vi "Top Level FPGA_w8LED.vi"() -> ()   [LabVIEW 2012]
uses:
  <vilib>/Platform/TimedLoop/XDataNode/timing_clust.ctl
  <vilib>/Platform/TimedLoop/XDataNode/nitl_modes.ctl
  <vilib>/Platform/TimedLoop/XDataNode/wakeup.ctl
  <vilib>/rvi/DataTransferAndStorage/Container/Common/niFpgaContainerMetaDataKey.ctl
  <vilib>/rvi/DataTransferAndStorage/Container/Common/niFpgaContainerState.ctl
  <vilib>/rvi/DataTransferAndStorage/Container/Common/niFpgaDataTypeControl.ctl
  <vilib>/rvi/DataTransferAndStorage/Container/Common/niFpgaContainerImplementationControl.ctl
  <vilib>/rvi/DataTransferAndStorage/Container/Common/niFpgaContainerArbitrationOptionsControl.ctl
  <vilib>/rvi/DataTransferAndStorage/Container/Common/niFpgaTransferTypeControl.ctl
  <vilib>/rvi/DataTransferAndStorage/Container/Common/niFpgaContainerInitializationParameters.ctl
  <vilib>/rvi/Memory/Memory_Types/niFpgaMemoryInterfaceConfiguration.ctl
  <vilib>/rvi/FIFO/Fifo_Types/niFpgaFifoControlLogicControl.ctl
  <vilib>/rvi/eio/common/nirviEmuTemplateMethod_errors.vi
  <vilib>/rvi/FIFO/Fifo_Resource/nirvififoEmulationSetSize.vi
  <vilib>/rvi/DataTransferAndStorage/Container/Common/niFpgaContainerGetUniqueNameForEmu.vi
  <vilib>/rvi/Emulation/niFpgaSctlEmulationRegisterWithScheduler.vi
  <vilib>/rvi/Emulation/niFpgaSctlEmulationScheduler.vi
  <vilib>/rvi/Emulation/niFpgaSctlEmulationFifoFullMgr.vi
  <vilib>/rvi/errors/niFpgaSetErrorForExecOnDevCompSimple.vi
  <vilib>/rvi/eio/common/nirviEmuReportErrorAndStop.vi
  <vilib>/rvi/Memory/Memory_Emulation/nirvimemoryEmulationManagerCache_GetValue.vi
  <vilib>/rvi/Memory/Memory_Emulation/niFpgaMemoryEmulationValidateCache.vi
  <vilib>/rvi/Memory/Memory_Emulation/nirvimemoryEmulationManagerCache_InsertValue.vi
  <vilib>/rvi/Memory/Memory_Emulation/nirvimemoryEmulationManagerCache_SetValue.vi
  <vilib>/rvi/Emulation/niFpgaSctlEmulationResourceMgr.vi
  <vilib>/rvi/Memory/Memory_Emulation/niFpgaMemoryEmulationCacheClearOnFirstRun.vi
  <vilib>/rvi/Memory/Memory_Emulation/nirvimemoryEmulationManagerCache_MakeExclusive.vi
  <vilib>/rvi/Memory/Memory_Emulation/nirvimemoryEmulationManagerCache_ReleaseExclusive.vi
  <vilib>/Utility/error.llb/Clear Errors.vi
  <vilib>/rvi/DataTransferAndStorage/Container/Common/niFpgaContainerSetEmuInfo.vi
  <vilib>/eio/EIONode/EIONode.xnode
  <vilib>/Platform/TimedLoop/XDataNode/XDataNode.xnode
  <vilib>/rvi/DataTransferAndStorage/Container/XNode/niFpgaContainer.xnode
  <vilib>/rvi/FIFO/Fifo_Resource/nirvififoEmulationClear.vi
  <vilib>/rvi/FIFO/Fifo_Resource/nirvififoEmulationRead.vi
  <vilib>/rvi/DataTransferAndStorage/Register/Emulation/niFpgaRegisterEmulation.vi
  <vilib>/rvi/Memory/Memory_Emulation/nirvimemoryEmulation.vi
  <vilib>/rvi/FIFO/Fifo_Resource/nirvififoEmulationWrite.vi
  <vilib>/rvi/LocalResourceManager/LocalResourceManager.xnode
  <vilib>/Platform/TimedLoop/XDataNode/XDNodeRunTimeDep.lvlib
panel:
  out "IO Module\\ADC Error A":bool
  out "IO Module\\ADC Error B":bool
  out "IO Module\\Pll Unlocked":bool
  out "Exited cleanly?":bool
  in  "Stop FPGA and exit":bool
  in  "Record Size only data":u32=95
  in  "show_trigger_position_for_debugging":bool
  out "DMA FIFO Timed Out?":bool
  in  "circular buffer length":u32=1000
  in  "location":i16(ring) items=["Purdue", "NIKHEF", "Zurich", "???"]
  in  "Trigger 0":i16=4000
  in  "Trigger 1":i16=4000
  in  "Trigger 2":i16=4000
  in  "Trigger 3":i16=4000
  in  "Trigger 4":i16=4000
  in  "Trigger 5":i16=4000
  in  "Trigger 6":i16=4000
  in  "Trigger 7":i16=4000
  in  "# of pretrigger":u32=20
  in  "initial value":u64
  in  "channel 0 on/off":bool
  in  "channel 2 on/off":bool
  in  "channel 1 on/off":bool
  in  "channel 3 on/off":bool
  in  "channel 4 on/off":bool
  in  "channel 5 on/off":bool
  in  "channel 6 on/off":bool
  in  "channel 7 on/off":bool
  out "Is Channel 0 Test Pulse?":bool
  in  "Testpulse duration (20 ns ticks)":u32=1
  in  "Testpulse Separation (20 ns ticks)":u32=500
  in  "Testpulse Time Delay (20 ns ticks)":u32=15
  out "Timestamp":u64
  out "Is Channel 1 Test Pulse?":bool
  in  "Testpulser On/Off":bool
  out "Is Channel 2 Test Pulse?":bool
  out "Is Channel 3 Test Pulse?":bool
  out "Is Channel 4 Test Pulse?":bool
  out "Is Channel 5 Test Pulse?":bool
  out "Is Channel 6 Test Pulse?":bool
  out "Is Channel 7 Test Pulse?":bool
  out "Init Done":bool
  out "Initialize Flush DMA FIFO":bool
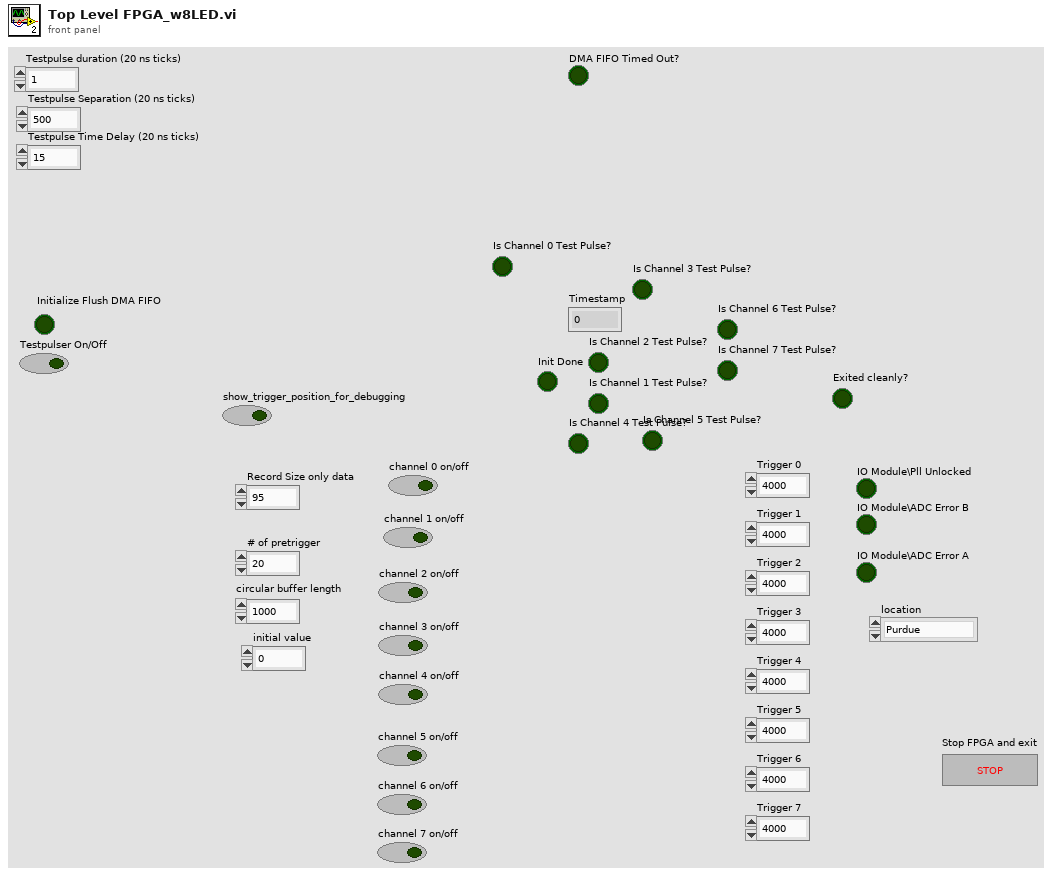
[diagram p1: front panel]
types:
  T1 = typedef "XDNodeRunTimeDep.lvlib/timing_clust.ctl" = cluster{"Expected End [f-1]":u64, "Actual End [f-1]":u64, "Finished Late? [f-1]":bool, "Expected End [i-1]":u64, "Actual End [i-1]":u64, "Finished Late? [i-1]":bool, "Expected Start [i]":u64, "Actual Start [i]":u64, "Expected Start [f]":u64, "Actual Start [f]":u64, "Source Name":string, "Structure Name":string, "Period":i64, "Deadline":i64, "Offset":i64, "Start":i64, "Priority":i32, "Timeout":i32, "Mode":T2, "Wakeup Reason":T3, "Error":errorcluster, "Source Type":string, "Secondary Source Type":string, "Global End Time":u64, "Global Start Time":u64, "Frame Duration":u64, "Iteration Duration":u64, "Assigned CPU":i32, "I/O Scan Engine Mode":u32}
  T2 = typedef "XDNodeRunTimeDep.lvlib/nitl_modes.ctl" = enum32{"No Change", "Process missed periods, maintain original phase", "Discard missed periods, maintain original phase", "Process missed periods, ignore original phase", "Discard missed periods, ignore original phase"}
  T3 = typedef "XDNodeRunTimeDep.lvlib/wakeup.ctl" = enum32{"Normal", "Aborted", "Asynchronous wakeup", "Timing source error", "Timed loop error", "Timeout"}
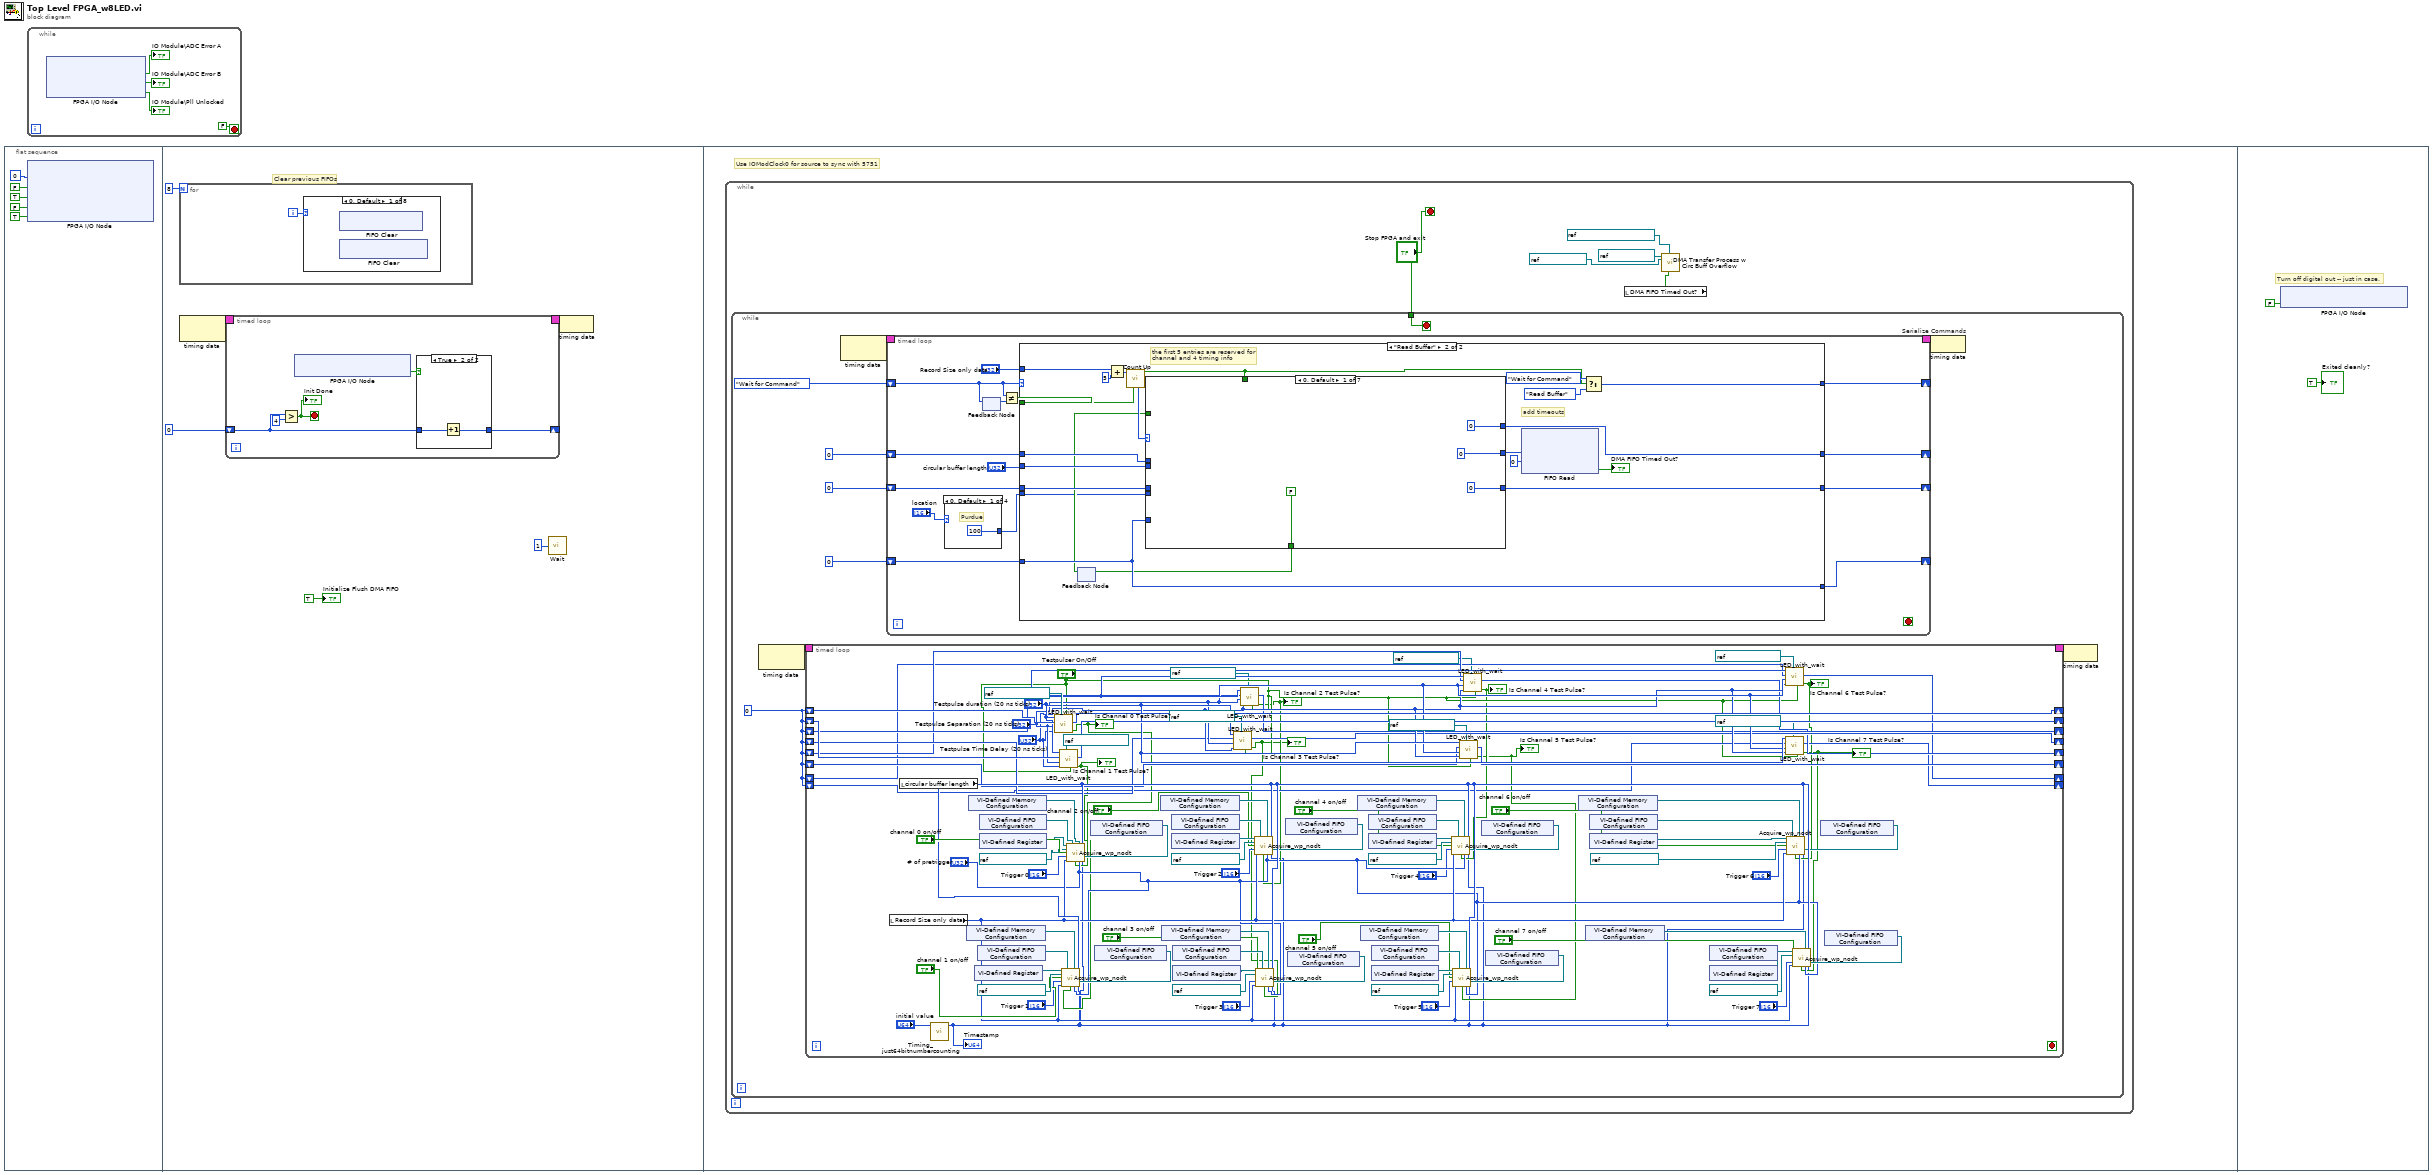
[diagram p0: block diagram]
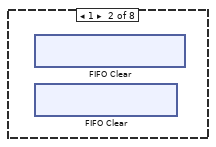
[diagram p2: hidden frame]
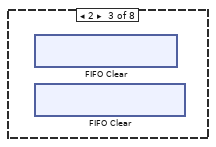
[diagram p3: hidden frame]
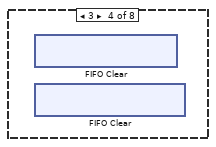
[diagram p4: hidden frame]
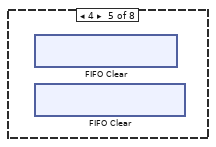
[diagram p5: hidden frame]
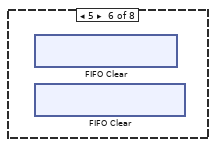
[diagram p6: hidden frame]
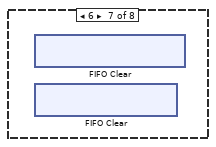
[diagram p7: hidden frame]
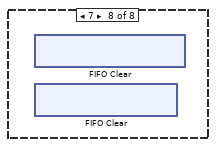
[diagram p8: hidden frame]
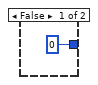
[diagram p9: hidden frame]
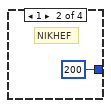
[diagram p10: hidden frame]
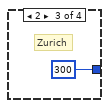
[diagram p11: hidden frame]
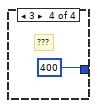
[diagram p12: hidden frame]
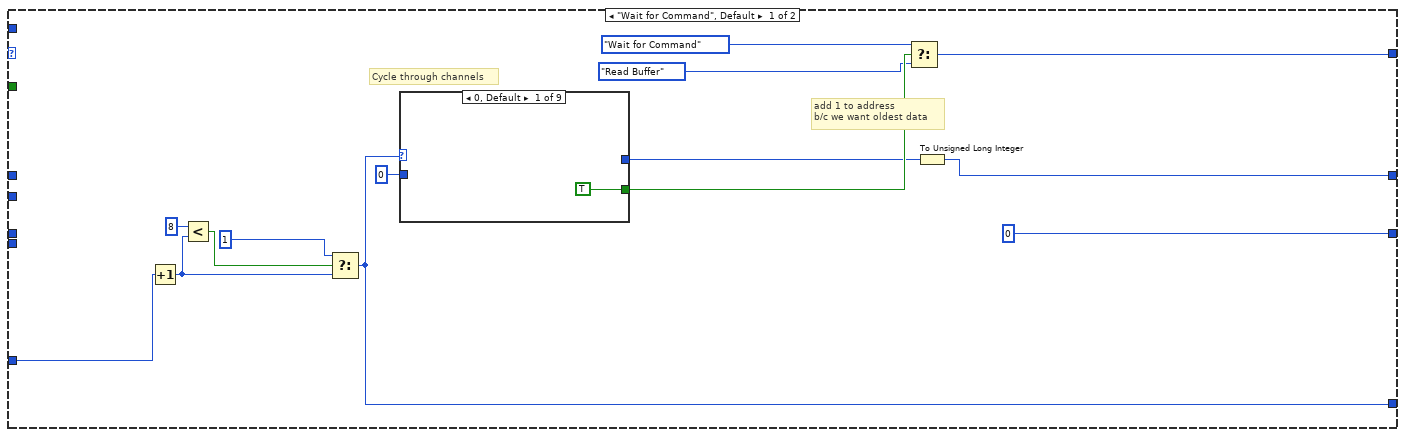
[diagram p13: hidden frame]
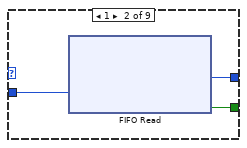
[diagram p14: hidden frame]
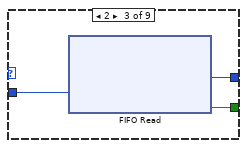
[diagram p15: hidden frame]
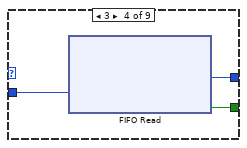
[diagram p16: hidden frame]
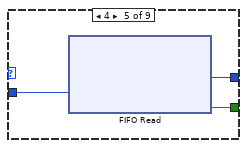
[diagram p17: hidden frame]
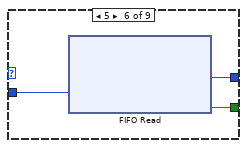
[diagram p18: hidden frame]
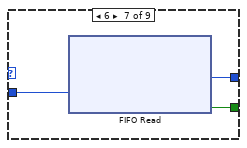
[diagram p19: hidden frame]
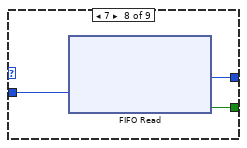
[diagram p20: hidden frame]
diagram:
  n1 = flat-sequence {
    frame #0 {
      n2 = xnode "FPGA I/O Node"("IO Module\\Sample Clock Select"=u8 0 ("IO Module\\Sample Clock Select"), "IO Module\\Force Initialization"=FALSE ("IO Module\\Force Initialization"), "IO Module\\Force Initialization"=TRUE ("IO Module\\Force Initialization"), "IO Module\\Force Initialization"=FALSE ("IO Module\\Force Initialization"), "IO Module\\Digital Output Enable"=TRUE ("IO Module\\Digital Output Enable")) -> ()  [unwired: 5 in, 5 out]
    }
    frame #1 {
      # "Clear previous FIFOs"
      n3 = for {
        N: 8 -> [_]
        i -> [w12]
        n4 = case shown="0, Default" w12 {
          frame 0, Default {
            n5 = xnode ("FIFO Clear")() -> ()  [unwired: 1 in, 1 out]
            n6 = xnode ("FIFO Clear")() -> ()  [unwired: 1 in, 1 out]
          }
          frame 1 {
            n7 = xnode ("FIFO Clear")() -> ()  [unwired: 1 in, 1 out]
            n8 = xnode ("FIFO Clear")() -> ()  [unwired: 1 in, 1 out]
          }
          frame 2 {
            n9 = xnode ("FIFO Clear")() -> ()  [unwired: 1 in, 1 out]
            n10 = xnode ("FIFO Clear")() -> ()  [unwired: 1 in, 1 out]
          }
          frame 3 {
            n11 = xnode ("FIFO Clear")() -> ()  [unwired: 1 in, 1 out]
            n12 = xnode ("FIFO Clear")() -> ()  [unwired: 1 in, 1 out]
          }
          frame 4 {
            n13 = xnode ("FIFO Clear")() -> ()  [unwired: 1 in, 1 out]
            n14 = xnode ("FIFO Clear")() -> ()  [unwired: 1 in, 1 out]
          }
          frame 5 {
            n15 = xnode ("FIFO Clear")() -> ()  [unwired: 1 in, 1 out]
            n16 = xnode ("FIFO Clear")() -> ()  [unwired: 1 in, 1 out]
          }
          frame 6 {
            n17 = xnode ("FIFO Clear")() -> ()  [unwired: 1 in, 1 out]
            n18 = xnode ("FIFO Clear")() -> ()  [unwired: 1 in, 1 out]
          }
          frame 7 {
            n19 = xnode ("FIFO Clear")() -> ()  [unwired: 1 in, 1 out]
            n20 = xnode ("FIFO Clear")() -> ()  [unwired: 1 in, 1 out]
          }
        }
      }
      n21 = node-c288() -> (w11:T1)  [unwired: 1 in]
      n22 = timed-loop {
        shift-right: [w16] -> _
        shift-left: u16 0 -> [w15]
        timing: w11 -> [_]
        timing-out: [_] -> w10
        stop <- w13 stop-if-true
        n23 = Greater?(x=w15, y=u16 4) -> (0:w13:bool)
        "Init Done" <- w13
        n24 = xnode "FPGA I/O Node"() -> ("IO Module\\Initialization Done"=w17:bool)  [unwired: 1 in, 1 out]
        n25 = case shown="True" w17 {
          tunnel: [u16 0 w20] -> w16
          tunnel: w15 -> [_ w19]
          frame False {
          }
          frame True {
            n26 = Increment(x=w19) -> (x+1=w20:u16)
          }
        }
      }
      n27 = call "Wait"("Count(mSec)"=u32 1) -> ()  [unwired: 1 out]
      n28 = node-c288(w10) -> ()
      "Initialize Flush DMA FIFO" <- TRUE ("Initialize Flush DMA FIFO")
    }
    frame #2 {
      # "Use IOModClock0 for source to sync with 5751"
      n29 = while {
        stop <- "Stop FPGA and exit" stop-if-true
        n30 = while {
          tunnel: "Stop FPGA and exit" -> [w31]
          stop <- w31 stop-if-true
          w30 = u64 0 ("Total number of pulses sent")
          n31 = node-c288() -> (w37:T1)  [unwired: 1 in]
          n32 = timed-loop {
            timing: w37 -> [_]
            timing-out: [_] -> w36
            shift-right: [w94] -> _
            shift-left: w30 -> [w95]
            shift-right: [w90] -> _
            shift-left: w30 -> [w91]
            shift-right: [w83] -> _
            shift-left: w30 -> [w84]
            shift-right: [w82] -> _
            shift-left: w30 -> [w77]
            shift-right: [w81] -> _
            shift-left: w30 -> [w76]
            shift-right: [w80] -> _
            shift-left: w30 -> [w75]
            shift-right: [w79] -> _
            shift-left: w30 -> [w74]
            shift-right: [w78] -> _
            shift-left: w30 -> [w73]
            stop <- _ stop-if-true
            n33 = local read "Record Size only data"() -> (w96:u32)
            n34 = local read "circular buffer length"() -> (w97:u32)
            n35 = call "Timing_just64bitnumbercounting.vi"("initial value"="initial value") -> ("x+1"=w40:u64)  [unwired: 10 in]
            "Timestamp" <- w40
            n36 = xnode "VI-Defined Memory Configuration"() -> ("Memory Out"=w136:refnum<k21>)
            n37 = xnode "VI-Defined Memory Configuration"() -> ("Memory Out"=w98:refnum<k21>)
            n38 = xnode "VI-Defined Register"() -> ("Register Out"=w88:refnum<k21>)
            n39 = xnode "VI-Defined FIFO Configuration"() -> ("FIFO Out"=w135:refnum<k21>)
            n40 = xnode "VI-Defined FIFO Configuration"() -> ("FIFO Out"=w99:refnum<k21>)
            n41 = xnode "VI-Defined Register"() -> ("Register Out"=w89:refnum<k21>)
            n42 = call "LED_with_wait.vi"("Testpulser On/Off"="Testpulser On/Off", "FPGA I/O In"=refnum<k21> "IO Module\\D0 0", "Testpulse Time Delay (20 ns ticks)"="Testpulse Time Delay (20 ns ticks)", "Testpulse Separation (20 ns ticks)"="Testpulse Separation (20 ns ticks)", "Total number of pulses input"=w95, "Testpulse duration (20 ns ticks)"="Testpulse duration (20 ns ticks)") -> ("Is Test Pulse?"=w42:bool, "Total number of pulses sent"=w94:u64)  [unwired: 4 in]
            "Is Channel 0 Test Pulse?" <- w42
            n43 = call "LED_with_wait.vi"("Testpulser On/Off"="Testpulser On/Off", "FPGA I/O In"=refnum<k21> "IO Module\\D0 1", "Testpulse Time Delay (20 ns ticks)"="Testpulse Time Delay (20 ns ticks)", "Testpulse Separation (20 ns ticks)"="Testpulse Separation (20 ns ticks)", "Total number of pulses input"=w91, "Testpulse duration (20 ns ticks)"="Testpulse duration (20 ns ticks)") -> ("Is Test Pulse?"=w41:bool, "Total number of pulses sent"=w90:u64)  [unwired: 4 in]
            "Is Channel 1 Test Pulse?" <- w41
            n44 = xnode "VI-Defined FIFO Configuration"() -> ("FIFO Out"=w65:refnum<k21>)
            n45 = call "Acquire_wp_nodt.vi"("Ch Armed Reg"=w89, "Command FIFO"=w99, "Circular Buffer Mem"=w98, "circular buffer length"=w97, "FPGA I/O In"=refnum<k21> "IO Module\\AI A0", "channel on/off"="channel 0 on/off", "Trigger"="Trigger 0", "Timing FIFO"=w65, "Samples to Acquire"=w96, "Is Test Pulse?"=w42, "# of pretrigger"="# of pretrigger", "timing"=w40) -> ()  [unwired: 4 in]
            n46 = xnode "VI-Defined FIFO Configuration"() -> ("FIFO Out"=w58:refnum<k21>)
            n47 = call "Acquire_wp_nodt.vi"("Ch Armed Reg"=w88, "Command FIFO"=w135, "Circular Buffer Mem"=w136, "circular buffer length"=w97, "FPGA I/O In"=refnum<k21> "IO Module\\AI A1", "channel on/off"="channel 1 on/off", "Trigger"="Trigger 1", "Timing FIFO"=w58, "Samples to Acquire"=w96, "Is Test Pulse?"=w41, "# of pretrigger"="# of pretrigger", "timing"=w40) -> ()  [unwired: 4 in]
            n48 = xnode "VI-Defined Memory Configuration"() -> ("Memory Out"=w132:refnum<k21>)
            n49 = xnode "VI-Defined Memory Configuration"() -> ("Memory Out"=w133:refnum<k21>)
            n50 = xnode "VI-Defined FIFO Configuration"() -> ("FIFO Out"=w131:refnum<k21>)
            n51 = xnode "VI-Defined Register"() -> ("Register Out"=w119:refnum<k21>)
            n52 = xnode "VI-Defined FIFO Configuration"() -> ("FIFO Out"=w134:refnum<k21>)
            n53 = xnode "VI-Defined Register"() -> ("Register Out"=w121:refnum<k21>)
            n54 = call "LED_with_wait.vi"("Testpulser On/Off"="Testpulser On/Off", "FPGA I/O In"=refnum<k21> "IO Module\\D0 3", "Testpulse Time Delay (20 ns ticks)"="Testpulse Time Delay (20 ns ticks)", "Testpulse Separation (20 ns ticks)"="Testpulse Separation (20 ns ticks)", "Total number of pulses input"=w77, "Testpulse duration (20 ns ticks)"="Testpulse duration (20 ns ticks)") -> ("Is Test Pulse?"=w43:bool, "Total number of pulses sent"=w82:u64)  [unwired: 4 in]
            "Is Channel 3 Test Pulse?" <- w43
            n55 = call "LED_with_wait.vi"("Testpulser On/Off"="Testpulser On/Off", "FPGA I/O In"=refnum<k21> "IO Module\\D0 2", "Testpulse Time Delay (20 ns ticks)"="Testpulse Time Delay (20 ns ticks)", "Testpulse Separation (20 ns ticks)"="Testpulse Separation (20 ns ticks)", "Total number of pulses input"=w84, "Testpulse duration (20 ns ticks)"="Testpulse duration (20 ns ticks)") -> ("Is Test Pulse?"=w44:bool, "Total number of pulses sent"=w83:u64)  [unwired: 4 in]
            "Is Channel 2 Test Pulse?" <- w44
            n56 = xnode "VI-Defined FIFO Configuration"() -> ("FIFO Out"=w64:refnum<k21>)
            n57 = call "Acquire_wp_nodt.vi"("Ch Armed Reg"=w119, "Command FIFO"=w131, "Circular Buffer Mem"=w132, "circular buffer length"=w97, "FPGA I/O In"=refnum<k21> "IO Module\\AI A2", "channel on/off"="channel 2 on/off", "Trigger"="Trigger 2", "Timing FIFO"=w64, "Samples to Acquire"=w96, "Is Test Pulse?"=w44, "# of pretrigger"="# of pretrigger", "timing"=w40) -> ()  [unwired: 4 in]
            n58 = xnode "VI-Defined FIFO Configuration"() -> ("FIFO Out"=w59:refnum<k21>)
            n59 = call "Acquire_wp_nodt.vi"("Ch Armed Reg"=w121, "Command FIFO"=w134, "Circular Buffer Mem"=w133, "circular buffer length"=w97, "FPGA I/O In"=refnum<k21> "IO Module\\AI A3", "channel on/off"="channel 3 on/off", "Trigger"="Trigger 3", "Timing FIFO"=w59, "Samples to Acquire"=w96, "Is Test Pulse?"=w43, "# of pretrigger"="# of pretrigger", "timing"=w40) -> ()  [unwired: 4 in]
            n60 = xnode "VI-Defined Memory Configuration"() -> ("Memory Out"=w124:refnum<k21>)
            n61 = xnode "VI-Defined Memory Configuration"() -> ("Memory Out"=w125:refnum<k21>)
            n62 = xnode "VI-Defined Register"() -> ("Register Out"=w113:refnum<k21>)
            n63 = xnode "VI-Defined FIFO Configuration"() -> ("FIFO Out"=w123:refnum<k21>)
            n64 = xnode "VI-Defined FIFO Configuration"() -> ("FIFO Out"=w126:refnum<k21>)
            n65 = xnode "VI-Defined Register"() -> ("Register Out"=w117:refnum<k21>)
            n66 = call "LED_with_wait.vi"("Testpulser On/Off"="Testpulser On/Off", "FPGA I/O In"=refnum<k21> "IO Module\\D0 5", "Testpulse Time Delay (20 ns ticks)"="Testpulse Time Delay (20 ns ticks)", "Testpulse Separation (20 ns ticks)"="Testpulse Separation (20 ns ticks)", "Total number of pulses input"=w75, "Testpulse duration (20 ns ticks)"="Testpulse duration (20 ns ticks)") -> ("Is Test Pulse?"=w45:bool, "Total number of pulses sent"=w80:u64)  [unwired: 4 in]
            "Is Channel 5 Test Pulse?" <- w45
            n67 = call "LED_with_wait.vi"("Testpulser On/Off"="Testpulser On/Off", "FPGA I/O In"=refnum<k21> "IO Module\\D0 4", "Testpulse Time Delay (20 ns ticks)"="Testpulse Time Delay (20 ns ticks)", "Testpulse Separation (20 ns ticks)"="Testpulse Separation (20 ns ticks)", "Total number of pulses input"=w76, "Testpulse duration (20 ns ticks)"="Testpulse duration (20 ns ticks)") -> ("Is Test Pulse?"=w46:bool, "Total number of pulses sent"=w81:u64)  [unwired: 4 in]
            "Is Channel 4 Test Pulse?" <- w46
            n68 = xnode "VI-Defined FIFO Configuration"() -> ("FIFO Out"=w63:refnum<k21>)
            n69 = call "Acquire_wp_nodt.vi"("Ch Armed Reg"=w113, "Command FIFO"=w123, "Circular Buffer Mem"=w124, "circular buffer length"=w97, "FPGA I/O In"=refnum<k21> "IO Module\\AI A4", "channel on/off"="channel 4 on/off", "Trigger"="Trigger 4", "Timing FIFO"=w63, "Samples to Acquire"=w96, "Is Test Pulse?"=w46, "# of pretrigger"="# of pretrigger", "timing"=w40) -> ()  [unwired: 4 in]
            n70 = xnode "VI-Defined FIFO Configuration"() -> ("FIFO Out"=w60:refnum<k21>)
            n71 = call "Acquire_wp_nodt.vi"("Ch Armed Reg"=w117, "Command FIFO"=w126, "Circular Buffer Mem"=w125, "circular buffer length"=w97, "FPGA I/O In"=refnum<k21> "IO Module\\AI A5", "channel on/off"="channel 5 on/off", "Trigger"="Trigger 5", "Timing FIFO"=w60, "Samples to Acquire"=w96, "Is Test Pulse?"=w45, "# of pretrigger"="# of pretrigger", "timing"=w40) -> ()  [unwired: 4 in]
            n72 = xnode "VI-Defined Memory Configuration"() -> ("Memory Out"=w129:refnum<k21>)
            n73 = xnode "VI-Defined Memory Configuration"() -> ("Memory Out"=w128:refnum<k21>)
            n74 = xnode "VI-Defined FIFO Configuration"() -> ("FIFO Out"=w130:refnum<k21>)
            n75 = xnode "VI-Defined Register"() -> ("Register Out"=w115:refnum<k21>)
            n76 = xnode "VI-Defined FIFO Configuration"() -> ("FIFO Out"=w127:refnum<k21>)
            n77 = xnode "VI-Defined Register"() -> ("Register Out"=w111:refnum<k21>)
            n78 = call "LED_with_wait.vi"("Testpulser On/Off"="Testpulser On/Off", "FPGA I/O In"=refnum<k21> "IO Module\\D0 6", "Testpulse Time Delay (20 ns ticks)"="Testpulse Time Delay (20 ns ticks)", "Testpulse Separation (20 ns ticks)"="Testpulse Separation (20 ns ticks)", "Total number of pulses input"=w74, "Testpulse duration (20 ns ticks)"="Testpulse duration (20 ns ticks)") -> ("Is Test Pulse?"=w48:bool, "Total number of pulses sent"=w79:u64)  [unwired: 4 in]
            "Is Channel 6 Test Pulse?" <- w48
            n79 = call "LED_with_wait.vi"("Testpulser On/Off"="Testpulser On/Off", "FPGA I/O In"=refnum<k21> "IO Module\\D0 7", "Testpulse Time Delay (20 ns ticks)"="Testpulse Time Delay (20 ns ticks)", "Testpulse Separation (20 ns ticks)"="Testpulse Separation (20 ns ticks)", "Total number of pulses input"=w73, "Testpulse duration (20 ns ticks)"="Testpulse duration (20 ns ticks)") -> ("Is Test Pulse?"=w47:bool, "Total number of pulses sent"=w78:u64)  [unwired: 4 in]
            "Is Channel 7 Test Pulse?" <- w47
            n80 = xnode "VI-Defined FIFO Configuration"() -> ("FIFO Out"=w62:refnum<k21>)
            n81 = call "Acquire_wp_nodt.vi"("Ch Armed Reg"=w115, "Command FIFO"=w130, "Circular Buffer Mem"=w129, "circular buffer length"=w97, "FPGA I/O In"=refnum<k21> "IO Module\\AI A6", "channel on/off"="channel 6 on/off", "Trigger"="Trigger 6", "Timing FIFO"=w62, "Samples to Acquire"=w96, "Is Test Pulse?"=w48, "# of pretrigger"="# of pretrigger", "timing"=w40) -> ()  [unwired: 4 in]
            n82 = xnode "VI-Defined FIFO Configuration"() -> ("FIFO Out"=w61:refnum<k21>)
            n83 = call "Acquire_wp_nodt.vi"("Ch Armed Reg"=w111, "Command FIFO"=w127, "Circular Buffer Mem"=w128, "circular buffer length"=w97, "FPGA I/O In"=refnum<k21> "IO Module\\AI A7", "channel on/off"="channel 7 on/off", "Trigger"="Trigger 7", "Timing FIFO"=w61, "Samples to Acquire"=w96, "Is Test Pulse?"=w47, "# of pretrigger"="# of pretrigger", "timing"=w40) -> ()  [unwired: 4 in]
          }
          n84 = node-c288() -> (w39:T1)  [unwired: 1 in]
          n85 = timed-loop "Serialize Commands" {
            timing: w39 -> [_]
            timing-out: [_] -> w38
            shift-right: [w917] -> _
            shift-left: enum16{"Wait for Command", "Read Buffer"}."Wait for Command" -> [w915]
            shift-right: [w921] -> _
            shift-left: u32 0 ("Element") -> [w920]
            shift-right: [w919] -> _
            shift-left: u8 0 ("t") -> [w918]
            shift-right: [w912] -> _
            shift-left: u64 0 ("Element") -> [w911]
            stop <- _ stop-if-true
            n86 = case shown="0, Default" "location" {
              tunnel: [i16 100 i16 200 i16 300 i16 400] -> w909
              frame 0, Default {
                # "Purdue"
              }
              frame 1 {
                # "NIKHEF"
              }
              frame 2 {
                # "Zurich"
              }
              frame 3 {
                # "???"
              }
            }
            n87 = feedback-in #1(w915) -> ()
            n88 = feedback #1() -> (w916:enum16{"Wait for Command", "Read Buffer"})  [unwired: 1 in]
            n89 = Not Equal?(x=w915, y=w916) -> (x != y?=w913:bool)
            n90 = case shown="\"Read Buffer\"" w915 {
              tunnel: "Record Size only data" -> [_ w975]
              tunnel: [w929 w985] -> w919
              tunnel: w918 -> [w931 w985]
              tunnel: [w932 w970] -> w921
              tunnel: w920 -> [_ w984]
              tunnel: [w935 w986] -> w917
              tunnel: "circular buffer length" -> [_ w983]
              tunnel: w913 -> [_ w977]
              tunnel: [u64 0 ("Element") w972] -> w912
              tunnel: w911 -> [_ w971]
              tunnel: w909 -> [_ w966]
              frame "Wait for Command", Default {
                # "add 1 to address\nb/c we want oldest data"
                # "Cycle through channels"
                n91 = Increment(x=w931) -> (x+1=w930:u8)
                n92 = Less?(x=u8 8, y=w930) -> (x < y?=w939:bool)
                n93 = Select(t=u8 1, s=w939, f=w930) -> (s? t:f=w929:u8)
                n94 = case shown="0, Default" w929 {
                  tunnel: [TRUE ("Timed Out?") w944 w945 w948 w951 w954 w957 w960 w963] -> w936
                  tunnel: 0 ("Timeout") -> [_ w943 w947 w950 w953 w956 w959 w962 w965]
                  tunnel: [_ w942 w946 w949 w952 w955 w958 w961 w964] -> w928
                  frame 0, Default {
                  }
                  frame 1 {
                    n95 = xnode ("FIFO Read")("Timeout"=w943) -> ("Element"=w942:i16, "Timed Out?"=w944:bool)  [unwired: 1 in, 1 out]
                  }
                  frame 2 {
                    n96 = xnode ("FIFO Read")("Timeout"=w947) -> ("Element"=w946:i16, "Timed Out?"=w945:bool)  [unwired: 1 in, 1 out]
                  }
                  frame 3 {
                    n97 = xnode ("FIFO Read")("Timeout"=w950) -> ("Element"=w949:i16, "Timed Out?"=w948:bool)  [unwired: 1 in, 1 out]
                  }
                  frame 4 {
                    n98 = xnode ("FIFO Read")("Timeout"=w953) -> ("Element"=w952:i16, "Timed Out?"=w951:bool)  [unwired: 1 in, 1 out]
                  }
                  frame 5 {
                    n99 = xnode ("FIFO Read")("Timeout"=w956) -> ("Element"=w955:i16, "Timed Out?"=w954:bool)  [unwired: 1 in, 1 out]
                  }
                  frame 6 {
                    n100 = xnode ("FIFO Read")("Timeout"=w959) -> ("Element"=w958:i16, "Timed Out?"=w957:bool)  [unwired: 1 in, 1 out]
                  }
                  frame 7 {
                    n101 = xnode ("FIFO Read")("Timeout"=w962) -> ("Element"=w961:i16, "Timed Out?"=w960:bool)  [unwired: 1 in, 1 out]
                  }
                  frame 8 {
                    n102 = xnode ("FIFO Read")("Timeout"=w965) -> ("Element"=w964:i16, "Timed Out?"=w963:bool)  [unwired: 1 in, 1 out]
                  }
                }
                n103 = Select(t=enum16{"Wait for Command", "Read Buffer"}."Wait for Command", s=w936, f=enum16{"Wait for Command", "Read Buffer"}."Read Buffer") -> (s? t:f=w935:enum16{"Wait for Command", "Read Buffer"})
                n104 = To Unsigned Long Integer(number=w928) -> (unsigned 32bit integer=w932:u32)
              }
              frame "Read Buffer" {
                # "the first 5 entries are reserved for channel and 4 timing info"
                # "add timeouts"
                n105 = feedback #2() -> (w969:bool)  [unwired: 1 in]
                n106 = Add(x=w975, y=u32 5) -> (x+y=w973:u32)
                n107 = call "Count Up.vi"("Reset?"=w977, "goal"=w973) -> ("Count Met"=w979:bool, "count"=w976:u32)  [unwired: 8 in]
                n108 = case shown="0, Default" w976 {
                  tunnel: w985 -> [_ w995 w1000 _ _ _ w1048]
                  tunnel: w984 -> [_ w999 w1002 w1032 w1038 w1044 w1055]
                  tunnel: w983 -> [_ _ _ _ _ _ w1054]
                  tunnel: w979 -> [_ _ _ _ _ _ w1053]
                  tunnel: [i16 0 ("Data") w996 w1006 w1030 w1036 w1042 w1049] -> w978
                  tunnel: w969 -> [_ _ _ _ _ _ w1051]
                  tunnel: [u64 0 ("Element") _ w1005 w1033 w1039 w1045 _] -> w972
                  tunnel: w971 -> [_ _ _ w1033 w1039 w1045 _]
                  tunnel: [u32 0 ("Element") w999 w1002 w1032 w1038 w1044 _] -> w970
                  tunnel: [FALSE FALSE FALSE FALSE FALSE TRUE FALSE] -> w968
                  tunnel: w966 -> [_ w991 _ _ _ _ _]
                  frame 0, Default {
                  }
                  frame 1 {
                    w997 = u16 0 items=["Header Information", "Particle Pulse", "Test Pulse"] ("Pulse Type")
                    n109 = Decrement(x=w995) -> (x-1=w994:u8)
                    n110 = To Word Integer(number=w994) -> (16bit integer=w993:i16)
                    n111 = Add(x=w991, y=w993) -> (x+y=w992:i16)
                    n112 = call "bitmanip.vi"("Pulse Type"=w997, "Integer to be written"=w992) -> ("Integer Written"=w996:i16)  [unwired: 2 in]
                  }
                  frame 2 {
                    n113 = case shown="1" w1000 {
                      tunnel: [_ w1007 w1009 w1011 w1013 w1015 w1017 w1019 w1021] -> w1001
                      frame Default {
                      }
                      frame 1 {
                        n114 = xnode ("FIFO Read")("Timeout"=0) -> ("Element"=w1007:u64)  [unwired: 1 in, 2 out]
                      }
                      frame 2 {
                        n115 = xnode ("FIFO Read")("Timeout"=0) -> ("Element"=w1009:u64)  [unwired: 1 in, 2 out]
                      }
                      frame 3 {
                        n116 = xnode ("FIFO Read")("Timeout"=0) -> ("Element"=w1011:u64)  [unwired: 1 in, 2 out]
                      }
                      frame 4 {
                        n117 = xnode ("FIFO Read")("Timeout"=0) -> ("Element"=w1013:u64)  [unwired: 1 in, 2 out]
                      }
                      frame 5 {
                        n118 = xnode ("FIFO Read")("Timeout"=0) -> ("Element"=w1015:u64)  [unwired: 1 in, 2 out]
                      }
                      frame 6 {
                        n119 = xnode ("FIFO Read")("Timeout"=0) -> ("Element"=w1017:u64)  [unwired: 1 in, 2 out]
                      }
                      frame 7 {
                        n120 = xnode ("FIFO Read")("Timeout"=0) -> ("Element"=w1019:u64)  [unwired: 1 in, 2 out]
                      }
                      frame 8 {
                        n121 = xnode ("FIFO Read")("Timeout"=0) -> ("Element"=w1021:u64)  [unwired: 1 in, 2 out]
                      }
                    }
                    n122 = case shown="True" "show_trigger_position_for_debugging" {
                      tunnel: [w1023 w1027] -> w1006
                      tunnel: [w1025 w1028] -> w1005
                      tunnel: w1002 -> [_ w1029]
                      tunnel: w1001 -> [w1025 w1028]
                      frame False {
                        # "reads out the lsb of the timing information"
                        n123 = Split Number(x=w1025) -> (hi(x)=w1026:u32)  [unwired: 1 out]
                        n124 = Split Number(x=w1026) -> (hi(x)=w1024:u16)  [unwired: 1 out]
                        n125 = To Word Integer(number=w1024) -> (16bit integer=w1023:i16)
                      }
                      frame True {
                        # "plot trigger position instead of the first timing bin"
                        n126 = To Word Integer(number=w1029) -> (16bit integer=w1027:i16)
                      }
                    }
                  }
                  frame 3 {
                    n127 = Split Number(x=w1033) -> (hi(x)=w1035:u32)  [unwired: 1 out]
                    n128 = Split Number(x=w1035) -> (lo(x)=w1034:u16)  [unwired: 1 out]
                    n129 = To Word Integer(number=w1034) -> (16bit integer=w1030:i16)
                  }
                  frame 4 {
                    n130 = Split Number(x=w1039) -> (lo(x)=w1041:u32)  [unwired: 1 out]
                    n131 = Split Number(x=w1041) -> (hi(x)=w1040:u16)  [unwired: 1 out]
                    n132 = To Word Integer(number=w1040) -> (16bit integer=w1036:i16)
                  }
                  frame 5 {
                    n133 = Split Number(x=w1045) -> (lo(x)=w1047:u32)  [unwired: 1 out]
                    n134 = Split Number(x=w1047) -> (lo(x)=w1046:u16)  [unwired: 1 out]
                    n135 = To Word Integer(number=w1046) -> (16bit integer=w1042:i16)
                  }
                  frame 6.. {
                    n136 = call "Circular Buffer Address_try_without_deadtime.vi"("Reset?"=w1051, "Starting Address"=w1055, "circular buffer length"=w1054) -> ("Address"=w1052:u32)  [unwired: 8 in]
                    n137 = case shown="Default" w1048 {
                      tunnel: w1052 -> [_ w1059 w1062 w1065 w1068 w1071 w1074 w1077 w1080]
                      tunnel: w1053 -> [_ w1058 w1061 w1064 w1067 w1070 w1073 w1076 w1079]
                      tunnel: [i16 0 w1057 w1060 w1063 w1066 w1069 w1072 w1075 w1078] -> w1049
                      frame Default {
                        # "Error"
                      }
                      frame 1 {
                        n138 = xnode ("Memory Read")("Address"=w1059) -> ("Data"=w1057:i16)  [unwired: 1 in, 1 out]
                        n139 = xnode ("Register Write")("Data"=w1058) -> ()  [unwired: 1 in, 1 out]
                      }
                      frame 2 {
                        n140 = xnode ("Memory Read")("Address"=w1062) -> ("Data"=w1060:i16)  [unwired: 1 in, 1 out]
                        n141 = xnode ("Register Write")("Data"=w1061) -> ()  [unwired: 1 in, 1 out]
                      }
                      frame 3 {
                        n142 = xnode ("Memory Read")("Address"=w1065) -> ("Data"=w1063:i16)  [unwired: 1 in, 1 out]
                        n143 = xnode ("Register Write")("Data"=w1064) -> ()  [unwired: 1 in, 1 out]
                      }
                      frame 4 {
                        n144 = xnode ("Memory Read")("Address"=w1068) -> ("Data"=w1066:i16)  [unwired: 1 in, 1 out]
                        n145 = xnode ("Register Write")("Data"=w1067) -> ()  [unwired: 1 in, 1 out]
                      }
                      frame 5 {
                        n146 = xnode ("Memory Read")("Address"=w1071) -> ("Data"=w1069:i16)  [unwired: 1 in, 1 out]
                        n147 = xnode ("Register Write")("Data"=w1070) -> ()  [unwired: 1 in, 1 out]
                      }
                      frame 6 {
                        n148 = xnode ("Memory Read")("Address"=w1074) -> ("Data"=w1072:i16)  [unwired: 1 in, 1 out]
                        n149 = xnode ("Register Write")("Data"=w1073) -> ()  [unwired: 1 in, 1 out]
                      }
                      frame 7 {
                        n150 = xnode ("Memory Read")("Address"=w1077) -> ("Data"=w1075:i16)  [unwired: 1 in, 1 out]
                        n151 = xnode ("Register Write")("Data"=w1076) -> ()  [unwired: 1 in, 1 out]
                      }
                      frame 8 {
                        n152 = xnode ("Memory Read")("Address"=w1080) -> ("Data"=w1078:i16)  [unwired: 1 in, 1 out]
                        n153 = xnode ("Register Write")("Data"=w1079) -> ()  [unwired: 1 in, 1 out]
                      }
                    }
                  }
                }
                n154 = feedback-in #2(w968) -> ()
                n155 = xnode ("FIFO Read")("Element"=w978, "Timeout"=0) -> ("Timed Out?"=→"DMA FIFO Timed Out?":bool)  [unwired: 1 in, 1 out]
                n156 = Select(t=enum16{"Wait for Command", "Read Buffer"}."Wait for Command", s=w979, f=enum16{"Wait for Command", "Read Buffer"}."Read Buffer") -> (s? t:f=w986:enum16{"Wait for Command", "Read Buffer"})
              }
            }
          }
          n157 = node-c288(w38) -> ()
          n158 = node-c288(w36) -> ()
        }
        n159 = local read "DMA FIFO Timed Out?"() -> (w26:bool)
        n160 = call "DMA Transfer Process w Circ Buff Overflow.vi"("DMA Write Timed Out?"=w26, "Clock Domain"=refnum<k21> "40 MHz Onboard Clock", "Local"=refnum<k21> "To DMA FIFO", "DMA"=refnum<k21> "To Host FIFO") -> ()  [unwired: 8 in]
      }
    }
    frame #3 {
      # "Turn off digital out -- just in case."
      n161 = xnode "FPGA I/O Node"("IO Module\\Digital Output Enable"=FALSE ("IO Module\\Digital Output Enable")) -> ()  [unwired: 1 in, 1 out]
      "Exited cleanly?" <- TRUE ("Exited cleanly?")
    }
  }
  n162 = while {
    stop <- FALSE stop-if-true
    n163 = xnode "FPGA I/O Node"() -> ("IO Module\\ADC Error A"=→"IO Module\\ADC Error A":bool, "IO Module\\ADC Error B"=→"IO Module\\ADC Error B":bool, "IO Module\\Pll Unlocked"=→"IO Module\\Pll Unlocked":bool)  [unwired: 3 in, 3 out]
  }
